vi "Next Step.vi"(8 "error in (no error)":errorcluster, 11 "Sequencer in":refnum<class "Sequencer.lvclass">) -> (0 "error out":errorcluster, 2 "Next Step":T1, 3 "Step Available":bool)   [LabVIEW 2020, in "Sequencer.lvclass"]
uses:
  Sequencer.lvclass
  Single Step Data.ctl
  Sequencer.lvclass/Sequencer.ctl
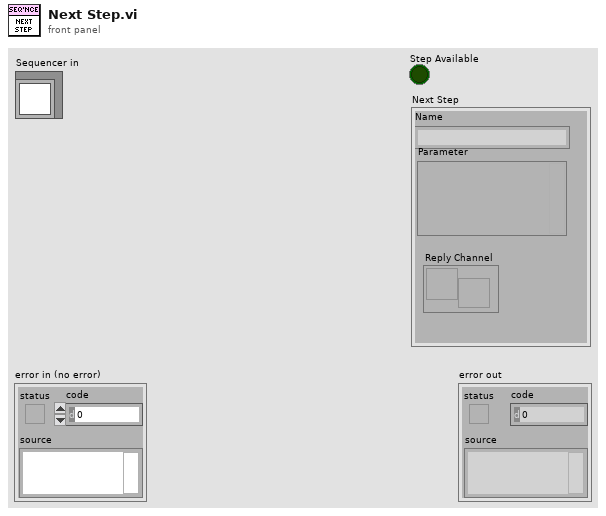
[diagram p1: front panel]
types:
  T1 = typedef "Sequencer.lvclass/Single Step Data.ctl" = cluster{"Name":string, "Parameter":variant, "Reply Channel":refnum<notifier>}
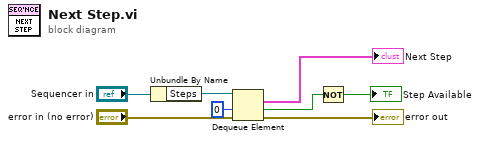
[diagram p0: block diagram]
diagram:
  n1 = Unbundle By Name("Sequencer in") -> ("Steps"=w4:refnum<queue>)
  n2 = Dequeue Element(queue=w4, timeout in ms (-1)=0, error in (no error)="error in (no error)") -> (element=→"Next Step":T1, timed out?=w5:bool, error out=→"error out":errorcluster)  [unwired: 1 out]
  n3 = Not(x=w5) -> (.not. x?=→"Step Available":bool)
